vi "SUB_DATETime_Convert.vi"(1 "Input SFCS DateTime String":string) -> (0 "DATE_TIME":string)   [LabVIEW 2011]
panel:
  out "SS":string
  out "MIN":string
  out "HR":string
  out "DAY":string
  out "MONTH":string
  out "YEAR":string
  out "after substring":string
  out "before substring":string
  # "因為SFCS 得到格式為 YEAR/Month/Day Hour:MIN:Seconds\n需轉換為 YEAR MONTH DAY HOUR MIN Seconds 給 Ubuntu Mojo Mobile"
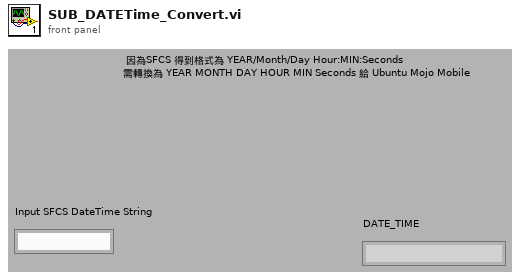
[diagram p1: front panel]
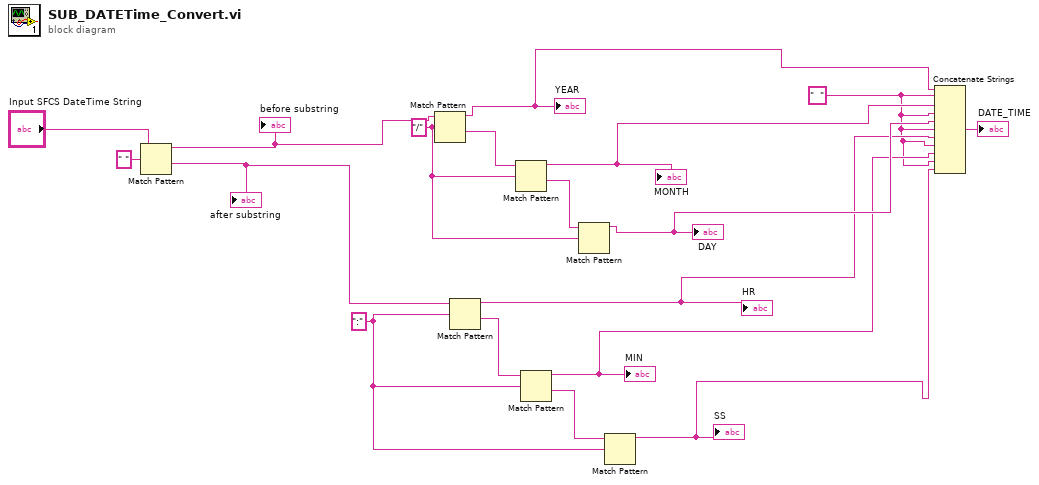
[diagram p0: block diagram]
diagram:
  w4 = "  " ("string")
  w10 = ":" ("regular expression")
  w14 = "/" ("regular expression")
  n1 = Match Pattern(string="Input SFCS DateTime String", regular expression=" ") -> (before substring=w17:string, after substring=w13:string)  [unwired: 1 in, 2 out]
  "before substring" <- w17
  "after substring" <- w13
  n2 = Match Pattern(string=w17, regular expression=w14) -> (before substring=w9:string, after substring=w16:string)  [unwired: 1 in, 2 out]
  "YEAR" <- w9
  n3 = Match Pattern(string=w13, regular expression=w10) -> (before substring=w6:string, after substring=w12:string)  [unwired: 1 in, 2 out]
  "HR" <- w6
  n4 = Match Pattern(string=w16, regular expression=w14) -> (before substring=w8:string, after substring=w15:string)  [unwired: 1 in, 2 out]
  "MONTH" <- w8
  n5 = Match Pattern(string=w12, regular expression=w10) -> (before substring=w5:string, after substring=w11:string)  [unwired: 1 in, 2 out]
  "MIN" <- w5
  n6 = Match Pattern(string=w15, regular expression=w14) -> (before substring=w7:string)  [unwired: 1 in, 3 out]
  "DAY" <- w7
  n7 = Match Pattern(string=w11, regular expression=w10) -> (before substring=w3:string)  [unwired: 1 in, 3 out]
  "SS" <- w3
  n8 = Concatenate Strings(w9, w4, w8, w4, w7, w4, w6, w4, w5, w4, w3) -> (→"DATE_TIME":string)
